vi "mb Convert [U16] to [U16].vi"(4 "U16":u16, 5 "U16 [ ]":u16[](array[numeric])) -> (1 "U16 [ ]":u16[](array[numeric]))   [LabVIEW 2009]
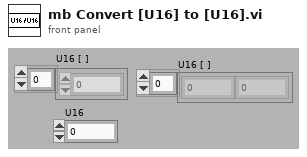
[diagram p1: front panel]
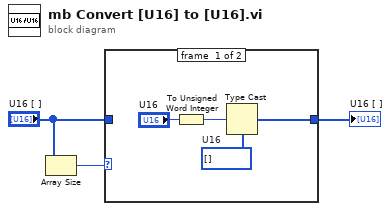
[diagram p0: block diagram]
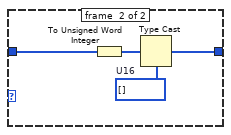
[diagram p2: hidden frame]
diagram:
  n1 = Array Size(array="U16 [ ]") -> (size(s)=w2:i32)
  n2 = case shown="Default" w2 {
    tunnel: "U16 [ ]" -> [_ w11]
    tunnel: [w4 w8] -> w1
    frame #0 {
      w6 = u16[] []  # U16
      n3 = To Unsigned Word Integer(number="U16") -> (unsigned 16bit integer=w7:u16)
      n4 = Type Cast(type=w6, x=w7) -> (*(type *) &x=w4:u16[])
    }
    frame #1 {
      w9 = u16[] []  # U16
      n5 = To Unsigned Word Integer(number=w11) -> (unsigned 16bit integer=w10:u16[])
      n6 = Type Cast(type=w9, x=w10) -> (*(type *) &x=w8:u16[])
    }
  }
  "U16 [ ]" <- w1
